vi "一体站流程自动启动.vi"(11 "参数":T1={"是否启用仪器"=FALSE, "CODMn"={"启动测量模式"={"测量模式"=enum."水样测量"}, "确定按钮"=TRUE}, "采水模式"=enum."使用采水泵"}) -> ()   [LabVIEW 2016, in "PLC.lvlib"]
uses:
  PLC.lvlib
panel:
  out "枚举":enum16{"初始化", "采配水启动", "等待", "配水", "排水", "结束"}(ring)
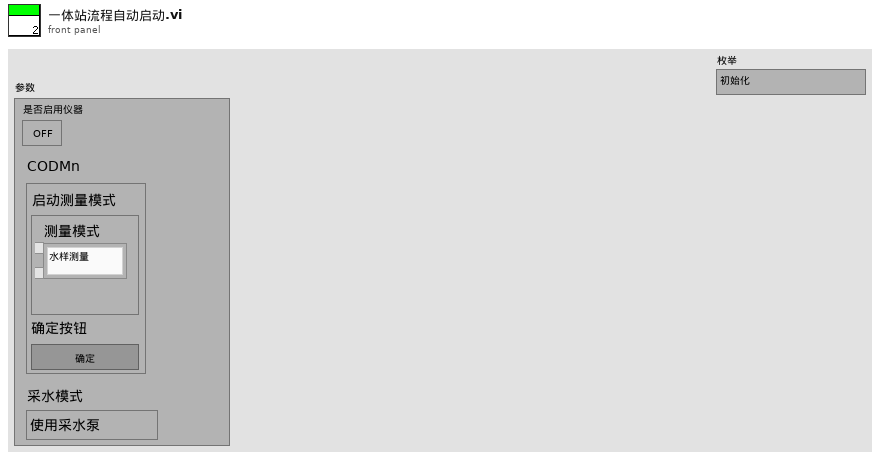
[diagram p1: front panel]
types:
  T1 = cluster{"是否启用仪器":bool, "CODMn":cluster{"启动测量模式":cluster{"测量模式":enum16{"水样测量", "标样核查", "零点核查", "加标回收", "平行样", "校零", "校标"}}, "确定按钮":bool}, "采水模式":enum16{"使用采水泵", "不使用采水泵"}}
  T2 = cluster{"命令":string, cluster{"starting address":u16, "holding register value":u16}}
  T3 = enum16{"待机", "启动氨氮", "氨氮测量中", "启动总磷", "总磷测量中", "结束"}
  T4 = cluster{"站号":u16, "量程切换":enum32{"H", "L", "AUTO"}, "控制命令":enum16{"启动测量", "标样核查", "零点核查", "跨度核查", "空白测试", "平行样测试", "加标回收", "空白校准", "标样校准", "初始化（清洗）", "停止测试", "仪器重启", "校时", "模式设置", "测量间隔设置", "盲样测试"}, "模式设置":enum16{"待机", "连续模式", "周期模式", "定点模式", "受控模式", "手动模式"}, "测量间隔":u16}
  T5 = cluster{"时间标识":timestamp, "设备":string, "日志信息":string}
  T6 = cluster{"测试时间":dbl, "运行模式":enum16{"维护模式", "常规模式", "应急模式", "质控模式"}}
  T7 = cluster{"R0":i16, "R1":i16, "R2":i16, "R3":i16, "R4":i16, "R5":i16, "R6":i16, "R7":i16, "R8":i16, "R9":i16, "R10":i16, "R11":i16, "R12":i16, "R13":i16, "R14":i16, "R15":i16, "R16":i16, "R17":i16, "R18":i16, "R19":i16, "R20":i16, "R21":i16}
  T8 = enum32{"Bad", "Idle", "Run top level", "Running"}
  T9 = cluster{"测量模式":enum16{"水样测量", "标样核查", "零点核查", "加标回收", "平行样", "校零", "校标"}}
  T10 = cluster{"系统时间":timestamp, "工作状态":enum16{"空闲", "水样测试", "标样核查", "零点核查", "跨度核查", "空白测试", "平行样测试", "加标回收", "空白校准", "标样校准", "初始化（清洗）"}, "测量模式":enum16{"待机", "连续模式", "周期模式", "定点模式", "受控模式", "手动模式"}, "告警代码":enum16{"无告警", "缺试剂告警", "缺水样告警", "缺蒸馏水告警", "缺标液告警", "仪表漏液告警", "标定异常告警", "超量程告警", "加热异常", "低试剂预警", "超上限告警", "超下限告警", "仪表内部其他异常", "滴定异常告警", "电极异常告警", "量程切换告警", "参数设置告警", "PH电极电位异常", "电导率电极异常", "浊度光度异常", "溶解氧电极异常", "溶解氧光强异常", "温度异常告警", "PH异常告警", "溶解氧异常告警", "电导率异常告警", "浊度异常告警", "叶绿素异常告警", "藻密度异常告警", "蓝绿藻异常告警", "ORP异常告警", "氨氮异常告警", "清洁刷异常告警", "SD卡异常告警", "蓝牙异常告警", "Wifi异常告警", "流程异常告警"}, "故障代码":enum16{"无故障", "电机故障", "温度故障", "通讯故障", "滴定故障"}, "日志代码":u16, "软件版本":u16, "F0":sgl, "F1":sgl, "F2":sgl, "F3":sgl, "T":sgl, "H":sgl, "id":u16, "flowid":u16, "量程":u16}
  T11 = enum16{"空闲", "水样测试", "标样核查", "零点核查", "跨度核查", "空白测试", "平行样测试", "加标回收", "空白校准", "标样校准", "初始化（清洗）"}
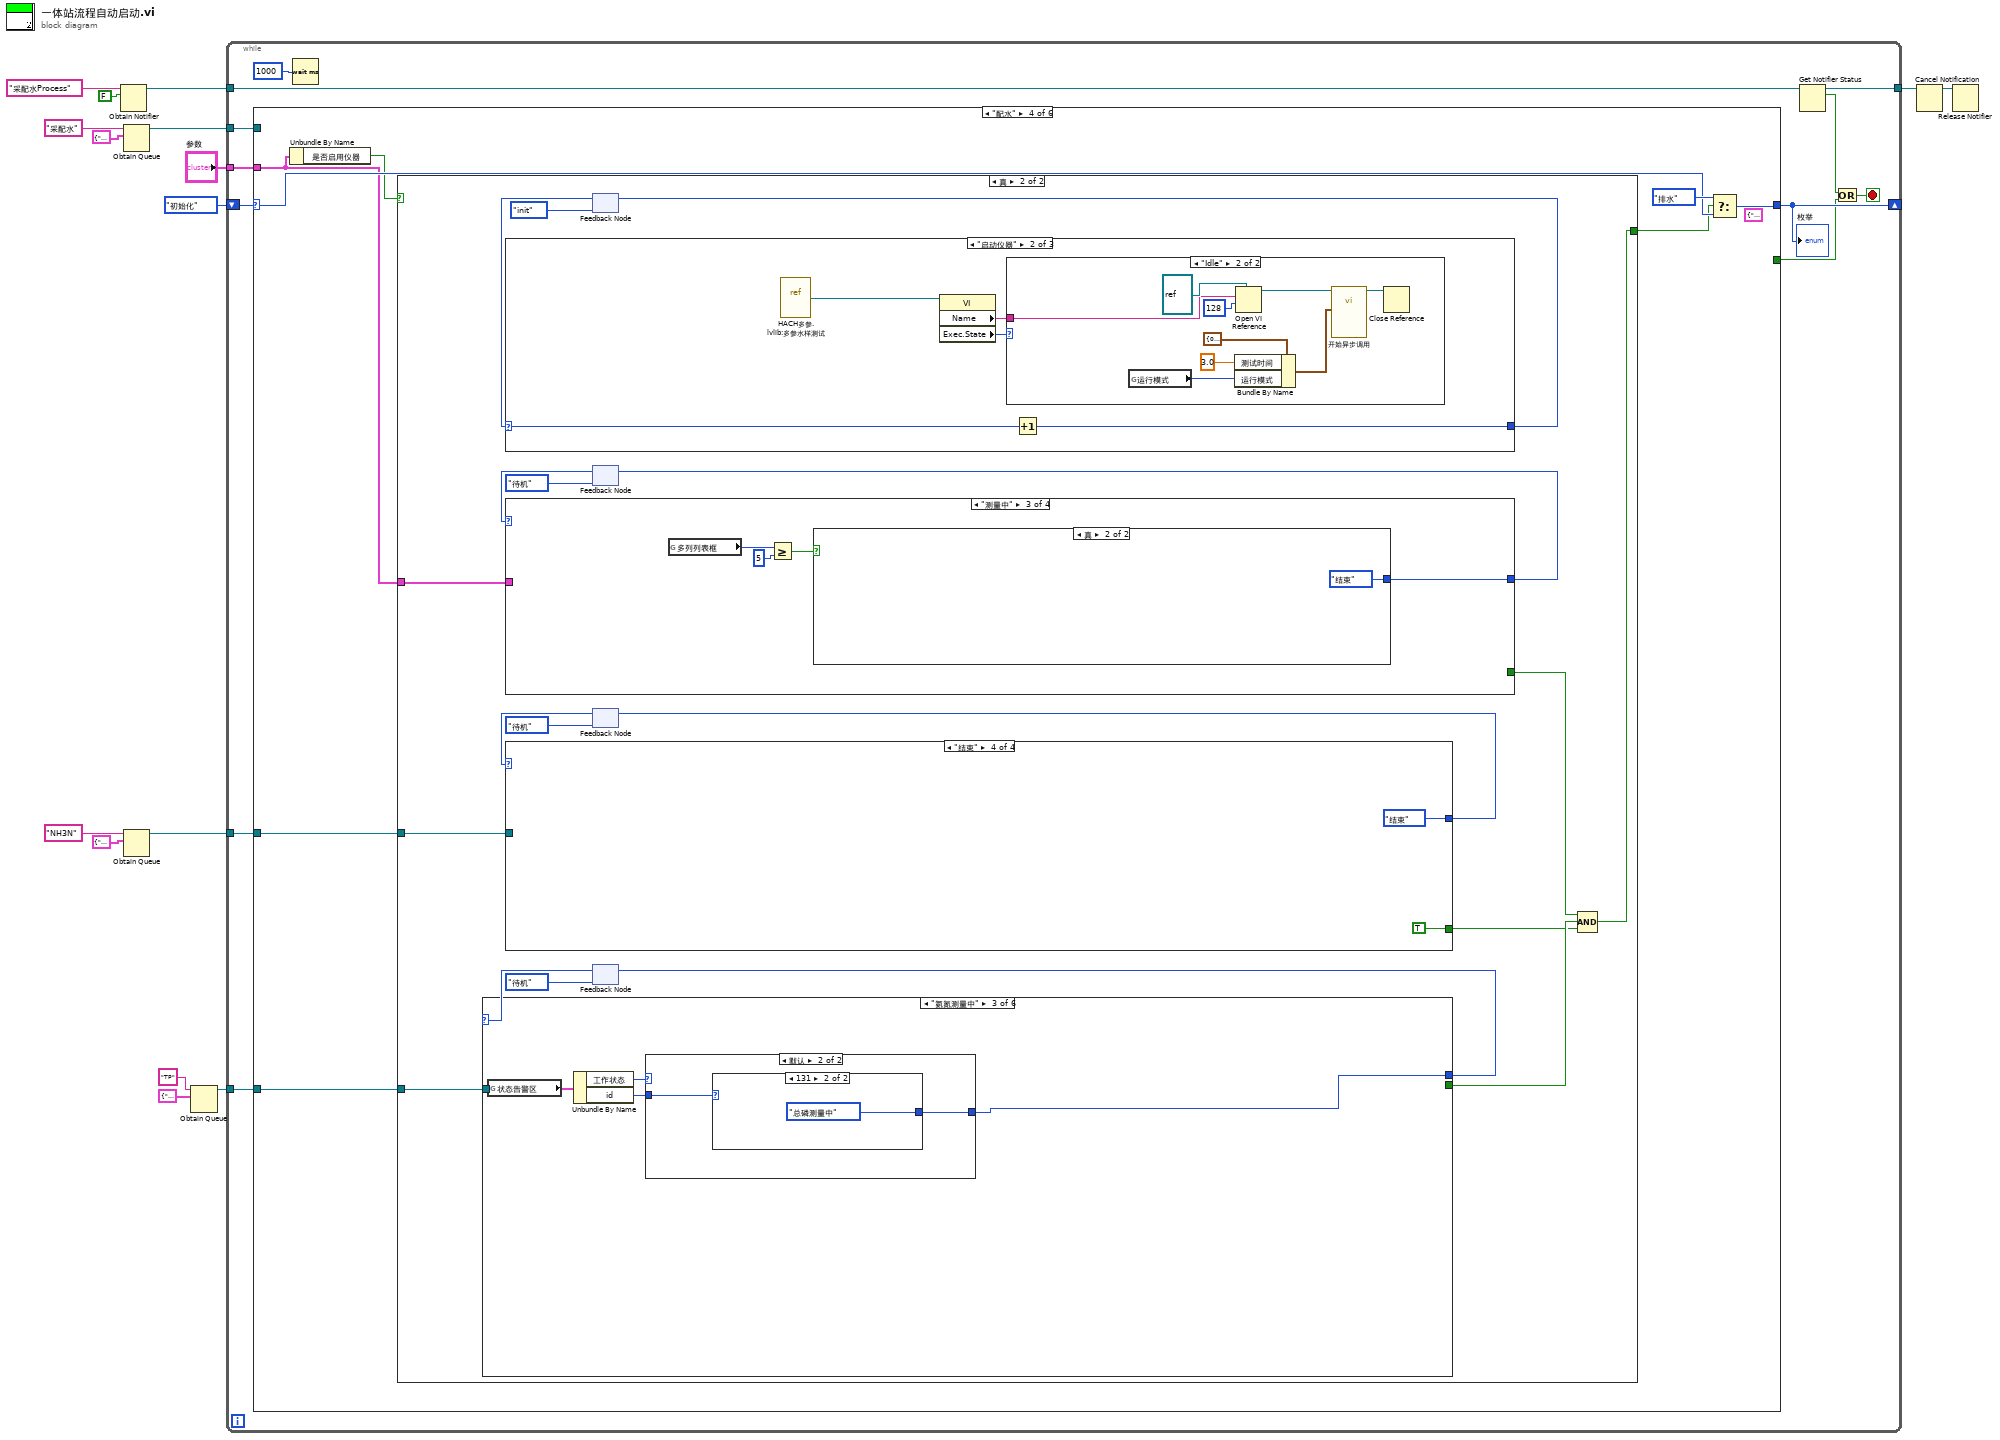
[diagram p0: block diagram]
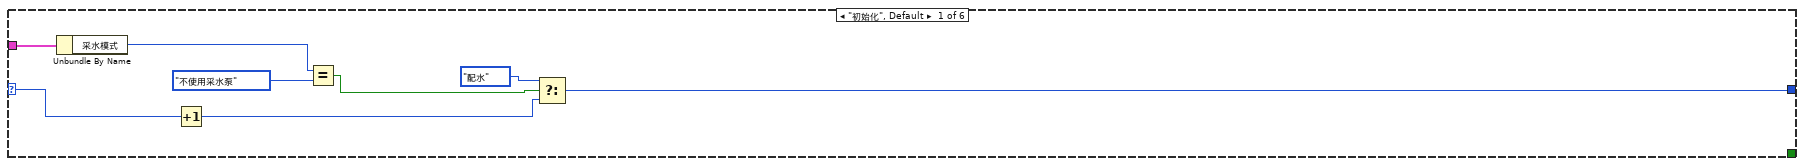
[diagram p2: hidden frame]
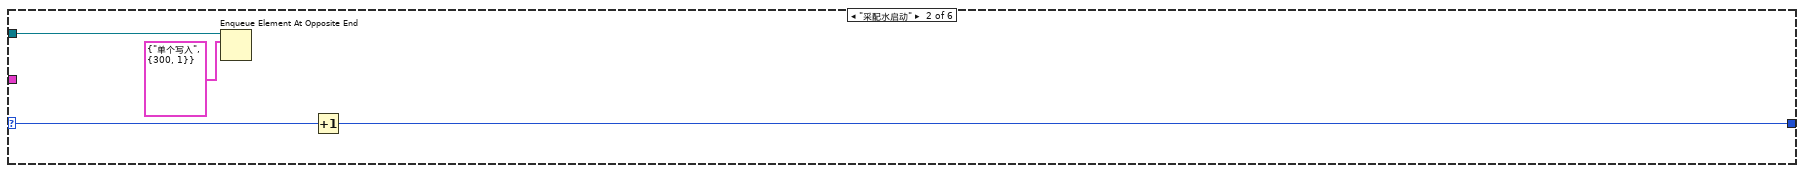
[diagram p3: hidden frame]
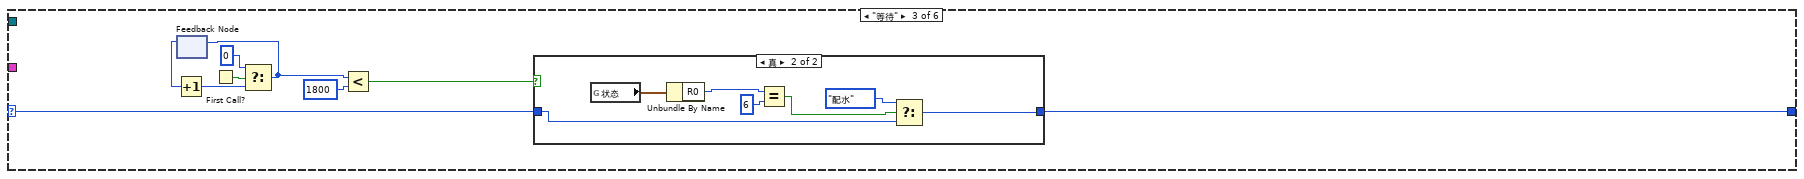
[diagram p4: hidden frame]
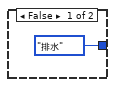
[diagram p5: hidden frame]
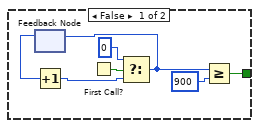
[diagram p6: hidden frame]
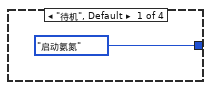
[diagram p7: hidden frame]
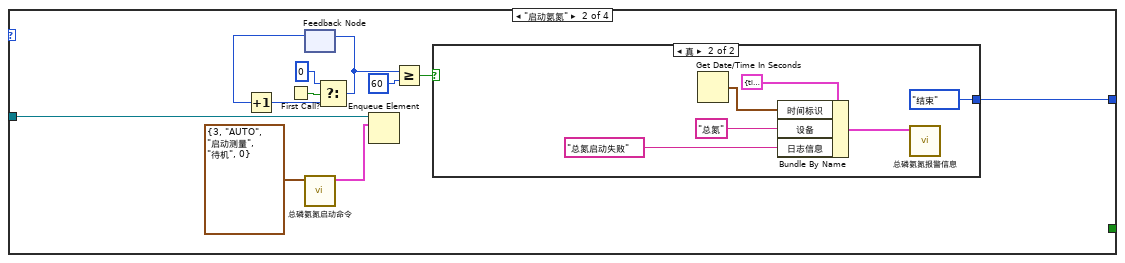
[diagram p8: hidden frame]
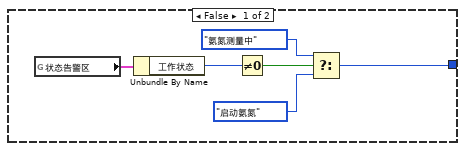
[diagram p9: hidden frame]
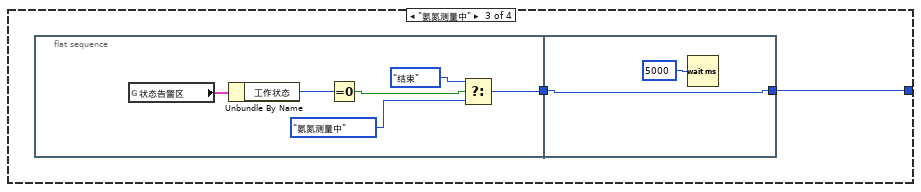
[diagram p10: hidden frame]
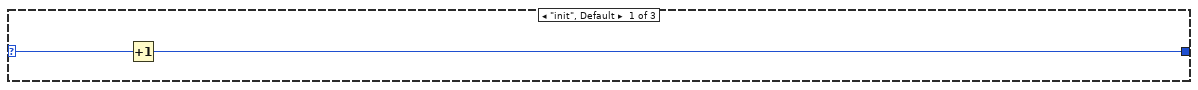
[diagram p11: hidden frame]
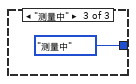
[diagram p13: hidden frame]
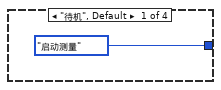
[diagram p14: hidden frame]
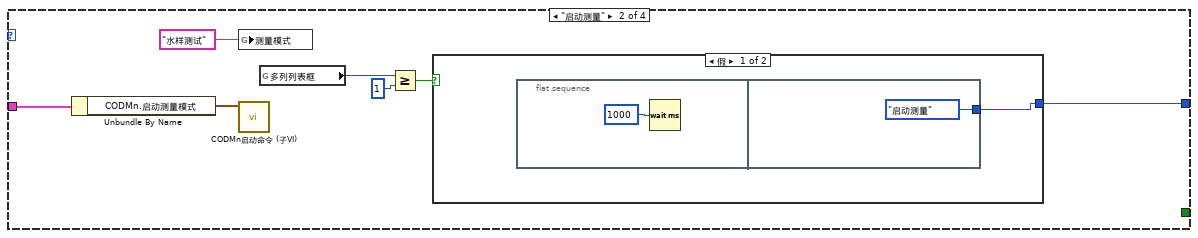
[diagram p15: hidden frame]
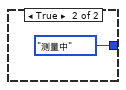
[diagram p16: hidden frame]
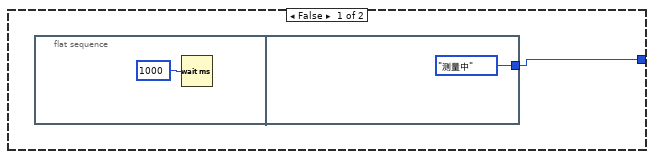
[diagram p17: hidden frame]
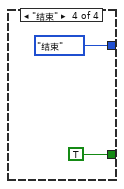
[diagram p18: hidden frame]
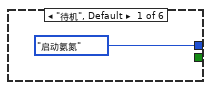
[diagram p19: hidden frame]
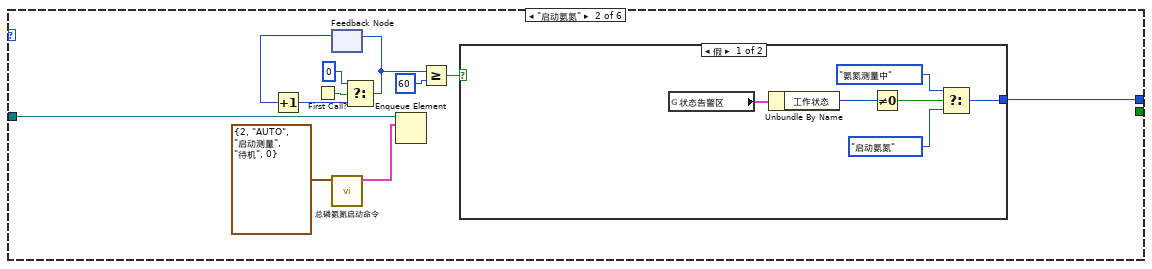
[diagram p20: hidden frame]
diagram:
  n1 = Obtain Notifier(name (unnamed)="采配水Process" ("名称（未命名）"), notification data type=FALSE) -> (notifier out=w6:refnum<notifier>)  [unwired: 2 in, 2 out]
  n2 = Obtain Queue(name (unnamed)="采配水" ("名称（未命名）"), element data type=cluster{"命令":string, "数据":variant} {"命令"="", "数据"=variant}) -> (queue out=w14:refnum<queue>)  [unwired: 3 in, 2 out]
  n3 = Obtain Queue(name (unnamed)="NH3N" ("名称（未命名）"), element data type=cluster{"命令":string, "data":variant} {"命令"="", "data"=variant}) -> (queue out=w1:refnum<queue>)  [unwired: 3 in, 2 out]
  n4 = Obtain Queue(name (unnamed)="TP" ("名称（未命名）"), element data type=cluster{"命令":string, "data":variant} {"命令"="", "data"=variant}) -> (queue out=w10:refnum<queue>)  [unwired: 3 in, 2 out]
  n5 = while {
    tunnel: w14 -> [w28]
    shift-right: [w26] -> _
    shift-left: enum16{"初始化", "采配水启动", "等待", "配水", "排水", "结束"}."初始化" ("枚举") -> [w27]
    tunnel: w10 -> [w24]
    tunnel: "参数" -> [w23]
    tunnel: w6 -> [w22]
    tunnel: [w21] -> w5
    tunnel: w1 -> [w17]
    stop <- w20 stop-if-true
    n6 = case shown="\"配水\"" w27 {
      selector: w27 -> [w36 w38 w47 w64 w237 w242]
      tunnel: w28 -> [_ w39 _ _ w238 _]
      tunnel: [w29 w37 w46 w63 w236 w241] -> w26
      tunnel: [_ _ _ _ _ TRUE] -> w19
      tunnel: w24 -> [_ _ _ w62 _ _]
      tunnel: w23 -> [w35 _ _ w59 _ _]
      tunnel: w17 -> [_ _ _ w58 _ _]
      frame "初始化", Default {
        n7 = Unbundle By Name(w35) -> ("采水模式"=w34:enum16{"使用采水泵", "不使用采水泵"})
        n8 = Increment(x=w36) -> (x+1=w30:enum16{"初始化", "采配水启动", "等待", "配水", "排水", "结束"})
        n9 = Equal?(x=w34, y=enum16{"使用采水泵", "不使用采水泵"}."不使用采水泵") -> (x = y?=w32:bool)
        n10 = Select(t=enum16{"初始化", "采配水启动", "等待", "配水", "排水", "结束"}."配水" ("枚举"), s=w32, f=w30) -> (s? t:f=w29:enum16{"初始化", "采配水启动", "等待", "配水", "排水", "结束"})
      }
      frame "采配水启动" {
        n11 = Enqueue Element At Opposite End(queue=w39, element=T2 {"命令"="单个写入", {"starting address"=300, "holding register value"=1}} ("元素")) -> ()  [unwired: 2 in, 3 out]
        n12 = Increment(x=w38) -> (x+1=w37:enum16{"初始化", "采配水启动", "等待", "配水", "排水", "结束"})
      }
      frame "等待" {
        n13 = feedback #1() -> (w43:i32)  [unwired: 1 in]
        n14 = Increment(x=w43) -> (x+1=w42:i32)
        n15 = First Call?() -> (First Call?: T/F=w44:bool)
        n16 = Select(t=0, s=w44, f=w42) -> (s? t:f=w41:i32)
        n17 = feedback-in #1(w41) -> ()
        n18 = Less?(x=w41, y=1800) -> (x < y?=w48:bool)
        n19 = case shown="真" w48 {
          tunnel: w47 -> [_ w52]
          tunnel: [enum16{"初始化", "采配水启动", "等待", "配水", "排水", "结束"}."排水" ("枚举") w51] -> w46
          frame False {
          }
          frame True {
            n20 = global read "采配水全局变量.vi" "状态"() -> (w57:T7)
            n21 = Unbundle By Name(w57) -> ("R0"=w56:i16)
            n22 = Equal?(x=w56, y=i16 6) -> (x = y?=w54:bool)
            n23 = Select(t=enum16{"初始化", "采配水启动", "等待", "配水", "排水", "结束"}."配水" ("枚举"), s=w54, f=w52) -> (s? t:f=w51:enum16{"初始化", "采配水启动", "等待", "配水", "排水", "结束"})
          }
        }
      }
      frame "配水" {
        (unwired) cluster{"命令":string, "data":variant} {"命令"="启动", "data"=variant(cluster{"站号":u16, "控制命令输出":u16[]} {"站号"=1, "控制命令输出"=[256, 0]})} ("元素")
        n24 = Unbundle By Name(w59) -> ("是否启用仪器"=w61:bool)
        n25 = case shown="真" w61 {
          tunnel: w62 -> [_ w88]
          tunnel: [w66 w73] -> w60
          tunnel: w59 -> [_ w84]
          tunnel: w58 -> [_ w77]
          frame False {
            n26 = feedback #2() -> (w70:i32)  [unwired: 1 in]
            n27 = Increment(x=w70) -> (x+1=w69:i32)
            n28 = First Call?() -> (First Call?: T/F=w71:bool)
            n29 = Select(t=0, s=w71, f=w69) -> (s? t:f=w67:i32)
            n30 = feedback-in #2(w67) -> ()
            n31 = Greater Or Equal?(x=w67, y=900) -> (x >= y?=w66:bool)
          }
          frame True {
            n32 = feedback #3(enum16{"init", "启动仪器", "测量中"}."init") -> (w82:enum16{"init", "启动仪器", "测量中"})
            n33 = case shown="\"启动仪器\"" w82 {
              selector: w82 -> [w129 w134 _]
              tunnel: [w128 w133 enum16{"init", "启动仪器", "测量中"}."测量中"] -> w83
              frame "init", Default {
                n34 = Increment(x=w129) -> (x+1=w128:enum16{"init", "启动仪器", "测量中"})
              }
              frame "启动仪器" {
                n35 = vi-ref "HACH多参.lvlib:多参水样测试.vi"() -> (w131:refnum<vi>)
                n36 = property class="VI"(reference=w131) -> ("Name"=w130:string, "Exec.State"=w132:T8)  [unwired: 1 in, 2 out]
                n37 = case shown="\"Idle\"" w132 {
                  tunnel: w130 -> [_ w141]
                  frame "Bad", Default {
                  }
                  frame "Idle" {
                    n38 = global read "系统变量.vi" "运行模式"() -> (w135:enum16{"维护模式", "常规模式", "应急模式", "质控模式"})
                    n39 = Bundle By Name(cluster=T6 {"测试时间"=0.0, "运行模式"=enum."维护模式"} ("API"), "测试时间"=3.0 ("测量时间"), "运行模式"=w135) -> (w137:T6)
                    n40 = Open VI Reference(type specifier VI Refnum (for type only)=refnum<vi> refnum ("类型说明符VI引用句柄（仅用于类型）"), vi path=w141, options=128 ("选项")) -> (vi reference=w140:refnum<vi>)  [unwired: 3 in, 1 out]
                    n41 = call-by-ref "开始异步调用"(reference=w140, "API"=w137) -> (reference out=w139:refnum<vi>)  [unwired: 12 in, 1 out]
                    n42 = Close Reference(reference=w139) -> ()  [unwired: 1 in, 1 out]
                  }
                }
                n43 = Increment(x=w134) -> (x+1=w133:enum16{"init", "启动仪器", "测量中"})
              }
              frame "测量中" {
              }
            }
            n44 = feedback-in #3(w83) -> ()
            n45 = feedback #4(enum16{"待机", "启动测量", "测量中", "结束"}."待机") -> (w86:enum16{"待机", "启动测量", "测量中", "结束"})
            n46 = case shown="\"测量中\"" w86 {
              tunnel: [enum16{"待机", "启动测量", "测量中", "结束"}."启动测量" w149 w158 enum16{"待机", "启动测量", "测量中", "结束"}."结束"] -> w85
              tunnel: w84 -> [_ w152 _ _]
              tunnel: [_ _ _ TRUE] -> w76
              frame "待机", Default {
              }
              frame "启动测量" {
                n47 = Unbundle By Name(w152) -> ("CODMn.启动测量模式"=w147:T9)
                n48 = global write "COD测量模式全局.vi" "测量模式"("水样测试" ("测量模式")) -> ()
                n49 = call "CODMn启动命令 (子VI).vi"("启动测量模式"=w147) -> ()  [unwired: 11 in]
                n50 = global read "运行时序全局变量.vi" "多列列表框"() -> (w148:i32)
                n51 = Greater Or Equal?(x=w148, y=1) -> (x >= y?=w150:bool)
                n52 = case shown="假" w150 {
                  tunnel: [w153 enum16{"待机", "启动测量", "测量中", "结束"}."测量中"] -> w149
                  frame False {
                    n53 = flat-sequence {
                      tunnel: [enum16{"待机", "启动测量", "测量中", "结束"}."启动测量"] -> w153
                      frame #0 {
                        n54 = Wait (ms)(milliseconds to wait=u32 1000 ("等待时间（毫秒）")) -> ()  [unwired: 1 out]
                      }
                      frame #1 {
                      }
                    }
                  }
                  frame True {
                  }
                }
              }
              frame "测量中" {
                n55 = global read "运行时序全局变量.vi" "多列列表框"() -> (w157:i32)
                n56 = Greater Or Equal?(x=w157, y=5) -> (x >= y?=w159:bool)
                n57 = case shown="真" w159 {
                  tunnel: [w161 enum16{"待机", "启动测量", "测量中", "结束"}."结束"] -> w158
                  frame False {
                    n58 = flat-sequence {
                      tunnel: [enum16{"待机", "启动测量", "测量中", "结束"}."测量中"] -> w161
                      frame #0 {
                        n59 = Wait (ms)(milliseconds to wait=u32 1000 ("等待时间（毫秒）")) -> ()  [unwired: 1 out]
                      }
                      frame #1 {
                      }
                    }
                  }
                  frame True {
                  }
                }
              }
              frame "结束" {
              }
            }
            n60 = feedback-in #4(w85) -> ()
            n61 = feedback #5(T3."待机") -> (w79:T3)
            n62 = case shown="\"结束\"" w79 {
              tunnel: [T3."启动氨氮" w102 w117 T3."结束"] -> w80
              tunnel: w77 -> [_ w103 _ _]
              tunnel: [_ _ _ TRUE] -> w74
              frame "待机", Default {
              }
              frame "启动氨氮" {
                n63 = First Call?() -> (First Call?: T/F=w100:bool)
                n64 = feedback #6() -> (w99:i32)  [unwired: 1 in]
                n65 = Increment(x=w99) -> (x+1=w98:i32)
                n66 = call "总磷氨氮启动命令.vi"("参数"=T4 {"站号"=3, "量程切换"=enum."AUTO", "控制命令"=enum."启动测量", "模式设置"=enum."待机", "测量间隔"=0}) -> ("启动命令"=w94:cluster{"命令":string, "data":variant})  [unwired: 10 in]
                n67 = Select(t=0, s=w100, f=w98) -> (s? t:f=w97:i32)
                n68 = feedback-in #6(w97) -> ()
                n69 = Enqueue Element(queue=w103, element=w94) -> ()  [unwired: 2 in, 3 out]
                n70 = Greater Or Equal?(x=w97, y=60) -> (x >= y?=w95:bool)
                n71 = case shown="真" w95 {
                  tunnel: [w106 T3."结束"] -> w102
                  frame False {
                    n72 = global read "VAR总磷氨氮全局变量.vi" "状态告警区"() -> (w109:T10)
                    n73 = Unbundle By Name(w109) -> ("工作状态"=w108:T11)
                    n74 = Not Equal To 0?(x=w108) -> (x != 0?=w107:bool)
                    n75 = Select(t=T3."氨氮测量中", s=w107, f=T3."启动氨氮") -> (s? t:f=w106:T3)
                  }
                  frame True {
                    n76 = Get Date/Time In Seconds() -> (seconds since 1Jan1904=w114:timestamp)
                    n77 = Bundle By Name(cluster=T5 {"时间标识"=timestamp(0 s since 1904-01-01), "设备"="", "日志信息"=""} ("data in"), "时间标识"=w114, "设备"="总氮", "日志信息"="总氮启动失败") -> (w110:T5)
                    n78 = call "总磷氨氮报警信息.vi"("data in"=w110) -> ()  [unwired: 11 in]
                  }
                }
              }
              frame "氨氮测量中" {
                n79 = flat-sequence {
                  tunnel: [w121] -> w116
                  tunnel: [w125] -> w117
                  tunnel: w116 -> [w125]
                  frame #0 {
                    n80 = global read "VAR总磷氨氮全局变量.vi" "状态告警区"() -> (w122:T10)
                    n81 = Unbundle By Name(w122) -> ("工作状态"=w123:T11)
                    n82 = Equal To 0?(x=w123) -> (x = 0?=w120:bool)
                    n83 = Select(t=T3."结束", s=w120, f=T3."氨氮测量中") -> (s? t:f=w121:T3)
                  }
                  frame #1 {
                    n84 = Wait (ms)(milliseconds to wait=u32 5000 ("等待时间（毫秒）")) -> ()  [unwired: 1 out]
                  }
                }
              }
              frame "结束" {
              }
            }
            n85 = feedback-in #5(w80) -> ()
            n86 = feedback #7(T3."待机") -> (w90:T3)
            n87 = case shown="\"氨氮测量中\"" w90 {
              tunnel: [T3."启动氨氮" w177 w191 w210 w224 T3."结束"] -> w89
              tunnel: w88 -> [_ w178 _ w211 _ _]
              tunnel: [_ _ _ _ _ TRUE] -> w75
              frame "待机", Default {
              }
              frame "启动氨氮" {
                n88 = First Call?() -> (First Call?: T/F=w175:bool)
                n89 = feedback #8() -> (w174:i32)  [unwired: 1 in]
                n90 = Increment(x=w174) -> (x+1=w173:i32)
                n91 = call "总磷氨氮启动命令.vi"("参数"=T4 {"站号"=2, "量程切换"=enum."AUTO", "控制命令"=enum."启动测量", "模式设置"=enum."待机", "测量间隔"=0}) -> ("启动命令"=w169:cluster{"命令":string, "data":variant})  [unwired: 10 in]
                n92 = Select(t=0, s=w175, f=w173) -> (s? t:f=w172:i32)
                n93 = feedback-in #8(w172) -> ()
                n94 = Enqueue Element(queue=w178, element=w169) -> ()  [unwired: 2 in, 3 out]
                n95 = Greater Or Equal?(x=w172, y=60) -> (x >= y?=w170:bool)
                n96 = case shown="假" w170 {
                  tunnel: [w181 T3."启动总磷"] -> w177
                  frame False {
                    n97 = global read "VAR总磷氨氮全局变量.vi" "状态告警区"() -> (w184:T10)
                    n98 = Unbundle By Name(w184) -> ("工作状态"=w183:T11)
                    n99 = Not Equal To 0?(x=w183) -> (x != 0?=w182:bool)
                    n100 = Select(t=T3."氨氮测量中", s=w182, f=T3."启动氨氮") -> (s? t:f=w181:T3)
                  }
                  frame True {
                    n101 = Get Date/Time In Seconds() -> (seconds since 1Jan1904=w189:timestamp)
                    n102 = Bundle By Name(cluster=T5 {"时间标识"=timestamp(0 s since 1904-01-01), "设备"="", "日志信息"=""} ("data in"), "时间标识"=w189, "设备"="总氮", "日志信息"="总氮启动失败") -> (w185:T5)
                    n103 = call "总磷氨氮报警信息.vi"("data in"=w185) -> ()  [unwired: 11 in]
                  }
                }
              }
              frame "氨氮测量中" {
                n104 = global read "VAR总磷氨氮全局变量.vi" "状态告警区"() -> (w194:T10)
                n105 = Unbundle By Name(w194) -> ("工作状态"=w192:T11, "id"=w193:u16)
                n106 = case shown="默认" w192 {
                  tunnel: w193 -> [_ w198]
                  tunnel: [T3."启动总磷" w197] -> w191
                  frame "空闲" {
                    n107 = Wait (ms)(milliseconds to wait=u32 8000 ("等待时间（毫秒）")) -> ()  [unwired: 1 out]
                  }
                  frame Default {
                    n108 = case shown="131" w198 {
                      tunnel: [T3."氨氮测量中" T3."总磷测量中"] -> w197
                      frame 76, Default {
                      }
                      frame 131 {
                      }
                    }
                  }
                }
              }
              frame "启动总磷" {
                n109 = First Call?() -> (First Call?: T/F=w208:bool)
                n110 = feedback #9() -> (w207:i32)  [unwired: 1 in]
                n111 = Increment(x=w207) -> (x+1=w206:i32)
                n112 = call "总磷氨氮启动命令.vi"("参数"=T4 {"站号"=1, "量程切换"=enum."AUTO", "控制命令"=enum."启动测量", "模式设置"=enum."待机", "测量间隔"=0}) -> ("启动命令"=w202:cluster{"命令":string, "data":variant})  [unwired: 10 in]
                n113 = Select(t=0, s=w208, f=w206) -> (s? t:f=w205:i32)
                n114 = feedback-in #9(w205) -> ()
                n115 = Enqueue Element(queue=w211, element=w202) -> ()  [unwired: 2 in, 3 out]
                n116 = Greater Or Equal?(x=w205, y=60) -> (x >= y?=w203:bool)
                n117 = case shown="真" w203 {
                  tunnel: [w214 T3."结束"] -> w210
                  frame False {
                    n118 = global read "VAR总磷氨氮全局变量.vi" "状态告警区"() -> (w215:T10)
                    n119 = Unbundle By Name(w215) -> ("工作状态"=w216:T11)
                    n120 = Not Equal To 0?(x=w216) -> (x != 0?=w217:bool)
                    n121 = Select(t=T3."总磷测量中", s=w217, f=T3."启动总磷") -> (s? t:f=w214:T3)
                  }
                  frame True {
                    n122 = Get Date/Time In Seconds() -> (seconds since 1Jan1904=w223:timestamp)
                    n123 = Bundle By Name(cluster=T5 {"时间标识"=timestamp(0 s since 1904-01-01), "设备"="", "日志信息"=""} ("data in"), "时间标识"=w223, "设备"="总磷", "日志信息"="总磷启动失败") -> (w218:T5)
                    n124 = call "总磷氨氮报警信息.vi"("data in"=w218) -> ()  [unwired: 11 in]
                  }
                }
              }
              frame "总磷测量中" {
                n125 = global read "VAR总磷氨氮全局变量.vi" "状态告警区"() -> (w227:T10)
                n126 = Unbundle By Name(w227) -> ("工作状态"=w225:T11, "id"=w226:u16)
                n127 = case shown="\"空闲\"" w225 {
                  tunnel: w226 -> [_ w231]
                  tunnel: [T3."结束" w230] -> w224
                  frame "空闲" {
                    n128 = Wait (ms)(milliseconds to wait=u32 8000 ("等待时间（毫秒）")) -> ()  [unwired: 1 out]
                  }
                  frame Default {
                    n129 = case shown="131" w231 {
                      tunnel: [T3."氨氮测量中" T3."总磷测量中"] -> w230
                      frame 76, Default {
                      }
                      frame 131 {
                      }
                    }
                  }
                }
              }
              frame "结束" {
              }
            }
            n130 = feedback-in #7(w89) -> ()
            n131 = Compound Arithmetic op=AND ("复合运算")(w76, w75, w74) -> (w73:bool)
          }
        }
        n132 = Select(t=enum16{"初始化", "采配水启动", "等待", "配水", "排水", "结束"}."排水" ("枚举"), s=w60, f=w64) -> (s? t:f=w63:enum16{"初始化", "采配水启动", "等待", "配水", "排水", "结束"})
      }
      frame "排水" {
        n133 = Enqueue Element At Opposite End(queue=w238, element=T2 {"命令"="单个写入", {"starting address"=303, "holding register value"=1}} ("元素")) -> ()  [unwired: 2 in, 3 out]
        n134 = Increment(x=w237) -> (x+1=w236:enum16{"初始化", "采配水启动", "等待", "配水", "排水", "结束"})
      }
      frame "结束" {
        n135 = Increment(x=w242) -> (x+1=w241:enum16{"初始化", "采配水启动", "等待", "配水", "排水", "结束"})
      }
    }
    "枚举" <- w26
    n136 = Wait (ms)(milliseconds to wait=u32 1000 ("等待时间（毫秒）")) -> ()  [unwired: 1 out]
    n137 = Get Notifier Status(notifier=w22) -> (notifier out=w21:refnum<notifier>, current notification=w18:bool)  [unwired: 1 in, 3 out]
    n138 = Or(x=w18, y=w19) -> (x .or. y?=w20:bool)
  }
  n139 = Cancel Notification(0:w5) -> (8:w4:refnum<notifier>)  [unwired: 1 in, 2 out]
  n140 = Release Notifier(notifier=w4) -> ()  [unwired: 2 in, 3 out]
